vi "Shutdown.vi"(8 "Error In":errorcluster) -> (0 "Error Out":errorcluster)   [LabVIEW 2017, in "LabPack.lvlib"]
uses:
  LabPack.lvlib
  Private/Globals.vi
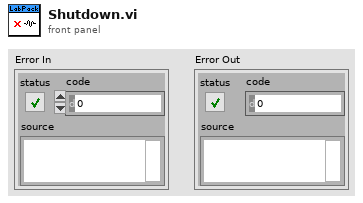
[diagram p1: front panel]
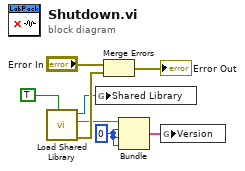
[diagram p0: block diagram]
diagram:
  w1 = u32 0
  n1 = call "Load Shared Library.vi"("Unload"=TRUE) -> ("Error Out"=w7:errorcluster, "Version"=w3:string, "LabPack Shared Library Out"=w4:path)  [unwired: 8 in]
  n2 = global write "Globals.vi" "Shared Library"(w4) -> ()
  n3 = Merge Errors("Error In", w7) -> (→"Error Out":errorcluster)
  n4 = Bundle("Version"=w3, w1, w1, w1) -> (w2:cluster{"Version":string, u32, u32, u32})  [unwired: 1 in]
  n5 = global write "Globals.vi" "Version"(w2) -> ()
